vi "Remove Client.vi"(8 "error in (no error)":errorcluster, 10 "Endpoint":string, 11 "Messaging Server Module in":refnum<class "Messaging Server Module.lvclass">) -> (0 "error out":errorcluster, 3 "Messaging Server Module out":refnum<class "Messaging Server Module.lvclass">)   [LabVIEW 2020, in "Volatus.lvlib" / "Messaging Server Module.lvclass"]
uses:
  Messaging Server Module.lvclass
  Messaging Server Module.lvclass/Messaging Server Module.ctl
  Msg Client State.ctl
  Volatus.lvlib
  Module/Module.lvclass
  VolatusAPI/VolatusAPI.lvclass
  Event Level.ctl
  C:/dev/lv20CE/relink/lv-volatus/Volatus/Module/Module.lvclass
  C:/dev/lv20CE/relink/lv-volatus/Volatus/Messaging Server Module/Messaging Server Module.lvclass
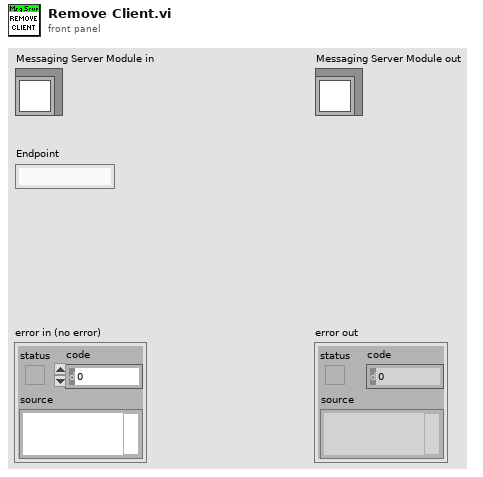
[diagram p1: front panel]
types:
  T1 = typedef "Volatus.lvlib/Msg Client State.ctl" = enum16{"Unknown", "Handshake", "Connected", "Closing"}
  T2 = typedef "Volatus.lvlib/Event Level.ctl" = enum16{"Debug", "Info", "Warning", "Error"}
  T3 = typedef "Volatus.lvlib/Messaging Server Module.lvclass/Client Info.ctl" = cluster{"MsgQ":refnum<class "MessageQ.lvclass">, "Address":string, "Port":u16, "Client State":T1, "Last Update":dbl, "Node":string, "Alias":string, "TCP":refnum<k5>}
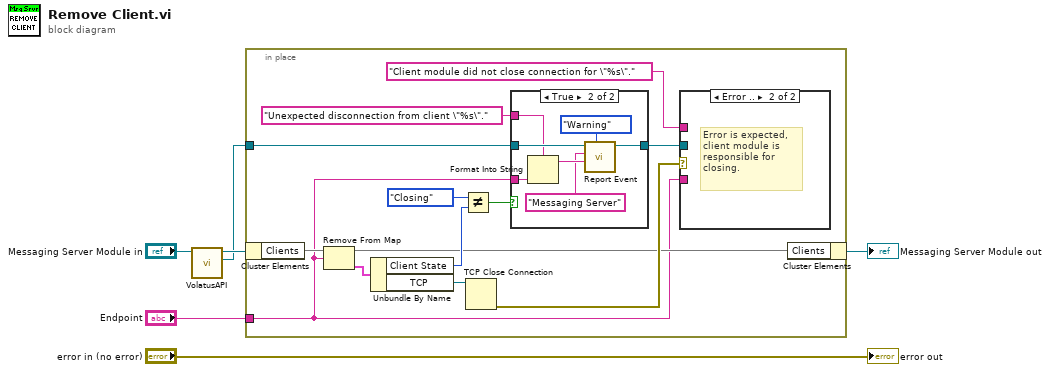
[diagram p0: block diagram]
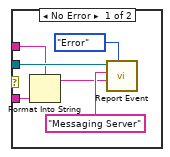
[diagram p2: hidden frame]
diagram:
  n1 = call "VolatusAPI.vi"("Module in"="Messaging Server Module in") -> ("VolatusAPI"=w2:refnum<class "VolatusAPI.lvclass">, "Module out"=w3:refnum<class "Messaging Server Module.lvclass">)  [unwired: 9 in]
  n2 = in-place {
    in-place-border: "Endpoint" -> [w8]
    in-place-border: w2 -> [w14]
    n3 = in-place-cluster #1(w3) -> ("Clients"=w18:map{string, T3})
    n4 = Remove From Map(10:w8, 11:w18) -> (1:w17:T3, 3:w13:map{string, T3})  [unwired: 1 out]
    n5 = Unbundle By Name(w17) -> ("Client State"=w16:T1, "TCP"=w10:refnum<k5>)
    n6 = Not Equal?(x=Msg_Client_State."Closing" ("y"), y=w16) -> (x != y?=w11:bool)
    n7 = TCP Close Connection(connection ID=w10) -> (error out=w19:errorcluster)  [unwired: 2 in, 1 out]
    n8 = case shown="True" w11 {
      tunnel: w14 -> [w26 w33]
      tunnel: "Unexpected disconnection from client \"%s\"." -> [_ w30]
      tunnel: w8 -> [_ w29]
      tunnel: [w26 w27] -> w9
      frame False {
      }
      frame True {
        n9 = Format Into String(format string=w30, w29) -> (resulting string=w31:string)  [unwired: 2 in, 1 out]
        n10 = call "Report Event.vi"("Level (Info)"=Event_Level."Warning", "Message"=w31, "Context"="Messaging Server", "VolatusAPI in"=w33) -> ("VolatusAPI out"=w27:refnum<class "VolatusAPI.lvclass">)  [unwired: 6 in, 1 out]
      }
    }
    n11 = case shown="Error .." w19 {
      tunnel: w9 -> [w25 _]
      tunnel: w8 -> [w22 _]
      tunnel: "Client module did not close connection for \"%s\"." -> [w21 _]
      frame No Error {
        n12 = Format Into String(format string=w21, w22) -> (resulting string=w20:string)  [unwired: 2 in, 1 out]
        n13 = call "Report Event.vi"("Level (Info)"=Event_Level."Error", "Message"=w20, "Context"="Messaging Server", "VolatusAPI in"=w25) -> ()  [unwired: 6 in, 2 out]
      }
      frame Error {
        # "Error is expected, client module is responsible for closing."
      }
    }
    n14 = in-place-cluster #1("Clients"=w13) -> (→"Messaging Server Module out":refnum<class "Messaging Server Module.lvclass">)
  }
  "error out" <- "error in (no error)"
